vi "SetPumpAlarms.vi"(0 "reference in":refnum<class "Stand.lvclass">, 11 "error in (no error)":errorcluster) -> (4 "reference out":refnum<class "Stand.lvclass">, 15 "error out":errorcluster)   [LabVIEW 2019, in "Stand.lvclass"]
uses:
  Stand.lvclass
  Engine_1DI_2DO_class/Engine_1DI_2DO.lvclass
  Engine_1DI_2DO_class/Config.ctl
  TypeDef/GUI Alarm developer settings.ctl
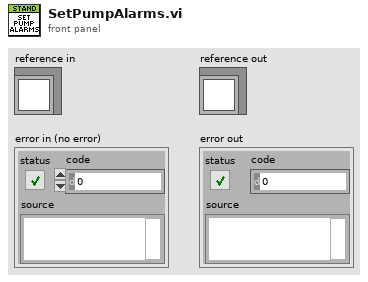
[diagram p1: front panel]
types:
  T1 = typedef "Engine_1DI_2DO.lvclass/Config.ctl" = cluster{"ON_TIMEOUT_MS":dbl, "OFF_TIMEOUT_MS":dbl}
  T2 = typedef "GUI Alarm developer settings.ctl" = cluster{"HIHI AI2":dbl, "HI AI2":dbl, "HIHI AI0":dbl, "HI AI0":dbl, "LOLO AI0":dbl, "LO AI0":dbl, "ENG2 OFF TIMEOUT":dbl, "ENG2 ON TIMEOUT":dbl, "HIHI AI3":dbl, "HI AI3":dbl, "HIHI AI1":dbl, "HI AI1":dbl, "LOLO AI1":dbl, "LO AI1":dbl, "ENG1 OFF TIMEOUT":dbl, "ENG1 ON TIMEOUT":dbl, "ENG0 OFF TIMEOUT":dbl, "ENG0 ON TIMEOUT":dbl, "LOLO AI8":dbl, "LO AI8":dbl, "LOLO AI9":dbl, "LO AI9":dbl, "LOLO AI5":dbl, "LO AI5":dbl, "Out Of Range HI":dbl, "Out Of Range LO":dbl}
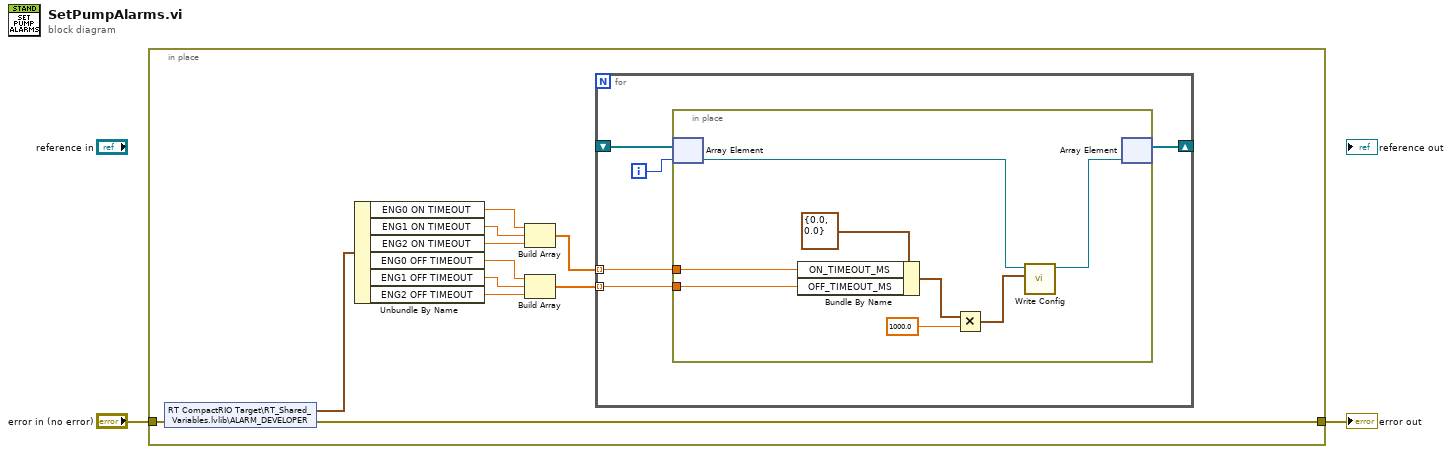
[diagram p0: block diagram]
diagram:
  n1 = in-place {
    in-place-border: "error in (no error)" -> [w15]
    in-place-border: [w14] -> w3
    n2 = shared-variable "RT CompactRIO Target\\RT_Shared_Variables.lvlib\\ALARM_DEVELOPER"(error in=w15) -> (w13:T2, error out=w14:errorcluster)
    n3 = Unbundle By Name(w13) -> ("ENG0 ON TIMEOUT"=w12:dbl, "ENG1 ON TIMEOUT"=w11:dbl, "ENG2 ON TIMEOUT"=w10:dbl, "ENG0 OFF TIMEOUT"=w9:dbl, "ENG1 OFF TIMEOUT"=w8:dbl, "ENG2 OFF TIMEOUT"=w7:dbl)
    n4 = Build Array(w12, w11, w10) -> (w6:dbl[])
    n5 = Build Array(w9, w8, w7) -> (w5:dbl[])
    n6 = for {
      shift-right: [w20] -> _
      shift-left: [w21] -> w16
      tunnel: w6 -> [w18] mode=indexing
      tunnel: w5 -> [w17] mode=indexing
      i -> [w19]
      n7 = in-place {
        in-place-border: w18 -> [w25]
        in-place-border: w17 -> [w24]
        n8 = in-place-array #1(w21, w19) -> (w29:refnum<class "Engine_1DI_2DO.lvclass">)
        n9 = Bundle By Name(cluster=T1 {"ON_TIMEOUT_MS"=0.0, "OFF_TIMEOUT_MS"=0.0} ("Config"), "ON_TIMEOUT_MS"=w25, "OFF_TIMEOUT_MS"=w24) -> (w26:T1)
        n10 = Multiply(x=w26, y=1000.0 ("ENG2 OFF TIMEOUT")) -> (x*y=w23:T1)
        n11 = call "Write Config.vi"("Config"=w23, "Pump_1AI_1DO_2DI in"=w29) -> ("Pump_1AI_1DO_2DI out"=w28:refnum<class "Engine_1DI_2DO.lvclass">)  [unwired: 9 in]
        n12 = in-place-array #1(w28) -> (w20:refnum<class "Engine_1DI_2DO.lvclass">[])  [unwired: 1 out]
      }
    }
  }
  "error out" <- w3
